vi "Differential Pressure Release Valve Test SAA.vi"(8 "error in (no error)":errorcluster, 10 "Model in":refnum<class "Model.lvclass">, 11 "Test Actuator State in":refnum<class "Test Actuator State.lvclass">) -> (0 "error out":errorcluster, 1 "Pass":bool, 2 "Model out":refnum<class "Model.lvclass">, 3 "Test Actuator State out":refnum<class "Test Actuator State.lvclass">)   [LabVIEW 2016, in "Test Actuator State.lvclass"]
uses:
  Test Actuator State.lvclass
  Model/Model/Model.lvclass
  Model/Model/Model.lvclass/Model.ctl
  Typedefs/ActuatorSetPoints.ctl
  <vilib>/Platform/TimedLoop/XDataNode/timing_clust.ctl
  <vilib>/Platform/TimedLoop/XDataNode/nitl_modes.ctl
  <vilib>/Platform/TimedLoop/XDataNode/wakeup.ctl
  <vilib>/platform/TimedLoop/XDataNode/XDataNode.xnode
  Typedefs/FAMT Typedefs.lvlib
  <vilib>/Platform/TimedLoop/XDataNode/XDNodeRunTimeDep.lvlib
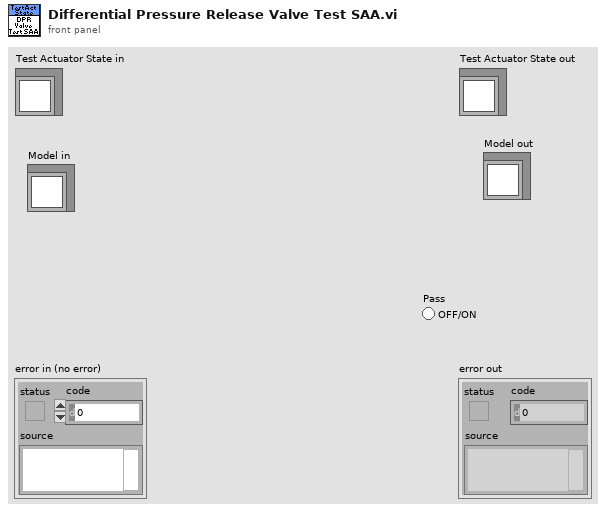
[diagram p1: front panel]
types:
  T1 = typedef "FAMT Typedefs.lvlib/DifferentialPressureReleaseValveTestSettings.ctl" = cluster{"Max Over Force (N)":dbl, "Max Moment (NM)":dbl, "Process Time (s)":dbl, "Sample Time (s)":dbl}
  T2 = typedef "FAMT Typedefs.lvlib/ForcePair.ctl" = cluster{"Axial Force":dbl, "Lateral Force":dbl}
  T3 = typedef "FAMT Typedefs.lvlib/FullForceScanSettings.ctl" = cluster{"Force Tolerance (N)":dbl, "DAA Force Set Points":T2[], "Process Time (s)":dbl, "Sample Time (s)":dbl, "Max Moment (NM)":dbl, "SAA Force Set Points":T2[]}
  T4 = typedef "FAMT Typedefs.lvlib/ActuatorSetPoints.ctl" = cluster{"Axial Force":dbl, "Lateral Force":dbl, "FC1 Force":dbl, "FC2 Force":dbl}
  T5 = typedef "XDNodeRunTimeDep.lvlib/timing_clust.ctl" = cluster{"Expected End [f-1]":u64, "Actual End [f-1]":u64, "Finished Late? [f-1]":bool, "Expected End [i-1]":u64, "Actual End [i-1]":u64, "Finished Late? [i-1]":bool, "Expected Start [i]":u64, "Actual Start [i]":u64, "Expected Start [f]":u64, "Actual Start [f]":u64, "Source Name":string, "Structure Name":string, "Period":i64, "Deadline":i64, "Offset":i64, "Start":i64, "Priority":i32, "Timeout":i32, "Mode":T6, "Wakeup Reason":T7, "Error":errorcluster, "Source Type":string, "Secondary Source Type":string, "Global End Time":u64, "Global Start Time":u64, "Frame Duration":u64, "Iteration Duration":u64, "Assigned CPU":i32, "I/O Scan Engine Mode":u32}
  T6 = typedef "XDNodeRunTimeDep.lvlib/nitl_modes.ctl" = enum32{"No Change", "Process missed periods, maintain original phase", "Discard missed periods, maintain original phase", "Process missed periods, ignore original phase", "Discard missed periods, ignore original phase"}
  T7 = typedef "XDNodeRunTimeDep.lvlib/wakeup.ctl" = enum32{"Normal", "Aborted", "Asynchronous wakeup", "Timing source error", "Timed loop error", "Timeout"}
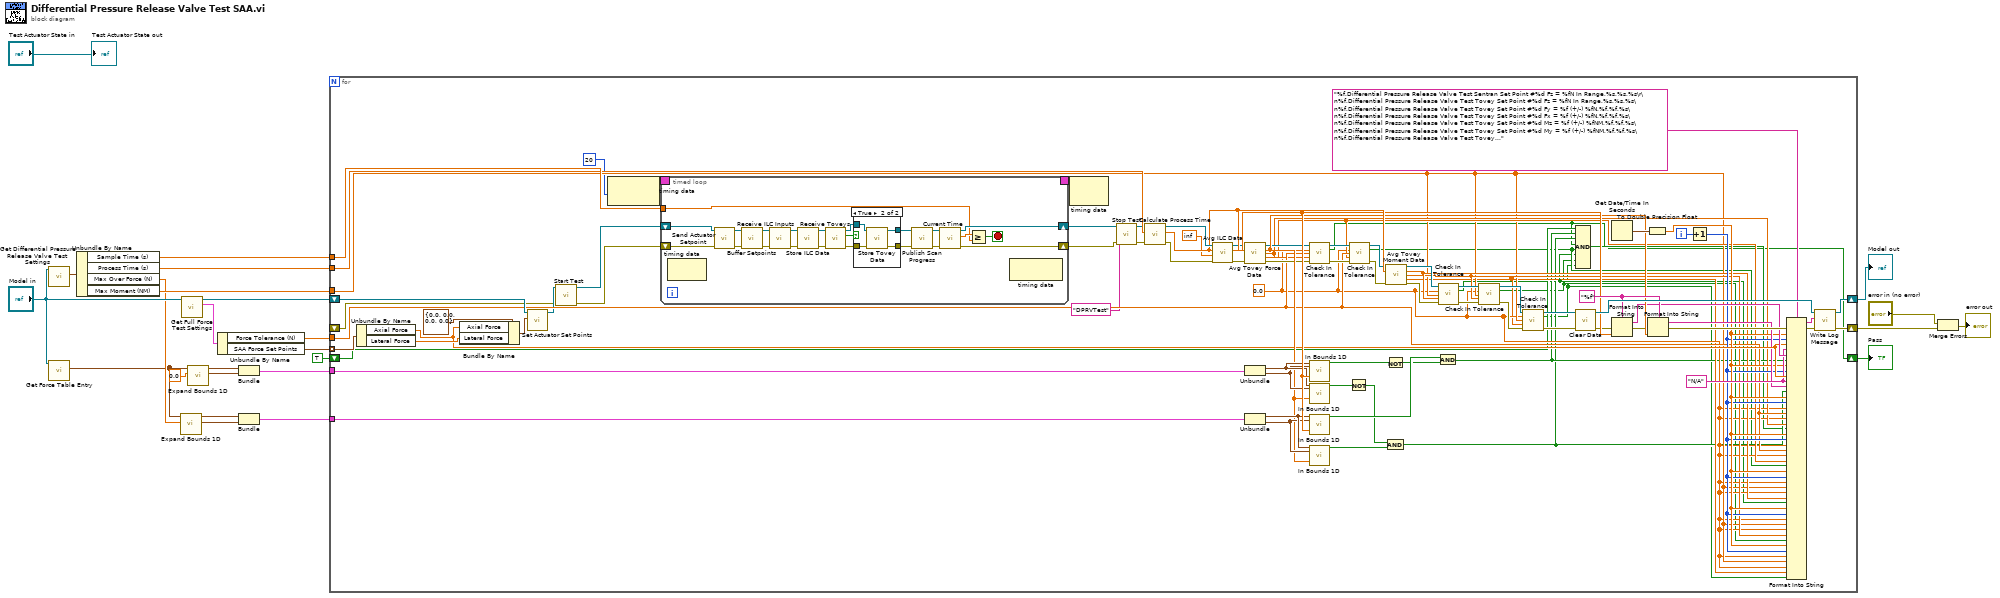
[diagram p0: block diagram]
diagram:
  n1 = call-dynamic "Get Differential Pressure Release Valve Test Settings.vi"("Model in"="Model in") -> ("Differential Pressure Release Valve Test Settings"=w14:T1)  [unwired: 9 in, 1 out]
  n2 = call "Get Force Table Entry.vi"("Model in"="Model in") -> ("Entry"=w8:T2[])  [unwired: 8 in, 2 out]
  n3 = Unbundle By Name(w14) -> ("Sample Time (s)"=w23:dbl, "Process Time (s)"=w22:dbl, "Max Over Force (N)"=w13:dbl, "Max Moment (NM)"=w17:dbl)
  n4 = call "Expand Bounds 1D.vi"("Tolerance (N)"=w13, "Entry"=w8) -> ("Bottom"=w10:T2, "Top"=w11:T2)  [unwired: 8 in]
  n5 = call "Get Full Force Test Settings.vi"("Model in"="Model in") -> ("Full Force Test Settings"=w16:T3, "Model out"=w24:refnum<class "Model.lvclass">)  [unwired: 9 in]
  n6 = call "Expand Bounds 1D.vi"("Tolerance (N)"=0.0, "Entry"=w8) -> ("Bottom"=w5:T2, "Top"=w6:T2)  [unwired: 8 in]
  n7 = Unbundle By Name(w16) -> ("Force Tolerance (N)"=w3:dbl, "SAA Force Set Points"=w12:T2[])
  n8 = Bundle("Top"=w6, "Bottom"=w5) -> (w4:cluster{"Top":T2, "Bottom":T2})  [unwired: 1 in]
  n9 = Bundle("Top"=w11, "Bottom"=w10) -> (w9:cluster{"Top":T2, "Bottom":T2})  [unwired: 1 in]
  n10 = for {
    tunnel: w12 -> [w104] mode=indexing
    shift-right: [w109] -> w19
    shift-left: w24 -> [w112]
    tunnel: w23 -> [w111]
    tunnel: w22 -> [w100]
    shift-right: [w101] -> w18
    shift-left: _ -> [w42]
    tunnel: w17 -> [w50]
    tunnel: w9 -> [w85]
    tunnel: w4 -> [w84]
    tunnel: w3 -> [w55]
    shift-right: [w27] -> w1
    shift-left: TRUE -> [w35]
    i -> [w106]
    w63 = "N/A" ("input 5")
    w79 = "%f" ("format string")
    w49 = 0.0
    n11 = Unbundle By Name(w104) -> ("Axial Force"=w64:dbl, "Lateral Force"=w80:dbl)
    n12 = Bundle By Name(cluster=T4 {"Axial Force"=0.0, "Lateral Force"=0.0, "FC1 Force"=0.0, "FC2 Force"=0.0} ("Actuator Set Points"), "Axial Force"=w64, "Lateral Force"=w80) -> (w105:T4)
    n13 = call "Set Actuator Set Points.vi"("Actuator Set Points"=w105, "Model in"=w112) -> ("Model out"=w43:refnum<class "Model.lvclass">)  [unwired: 9 in]
    n14 = call "Start Test.vi"("error in (no error)"=w42, "Model in"=w43) -> ("error out"=w41:errorcluster, "Model out"=w40:refnum<class "Model.lvclass">)  [unwired: 8 in]
    n15 = node-c288(i64 20 ("Period")) -> (w46:T5)
    n16 = timed-loop {
      shift-right: [w131] -> w39
      shift-left: w40 -> [w135]
      shift-right: [w130] -> w37
      shift-left: w41 -> [w133]
      tunnel: w111 -> [w128]
      timing: w46 -> [_]
      timing-out: [_] -> w45
      stop <- w127 stop-if-true
      n17 = node-c288() -> ()  [unwired: 1 in, 1 out]
      n18 = call "Send Actuator Setpoint.vi"("error in (no error)"=w133, "Model in"=w135) -> ("error out"=w115:errorcluster, "Model out"=w117:refnum<class "Model.lvclass">)  [unwired: 8 in]
      n19 = call "Buffer Setpoints.vi"("error in (no error)"=w115, "Model in"=w117) -> ("error out"=w114:errorcluster, "Model out"=w116:refnum<class "Model.lvclass">)  [unwired: 8 in]
      n20 = call "Receive ILC Inputs.vi"("error in (no error)"=w114, "Model in"=w116) -> ("error out"=w132:errorcluster, "Model out"=w134:refnum<class "Model.lvclass">)  [unwired: 8 in]
      n21 = call "Store ILC Data.vi"("error in (no error)"=w132, "Model in"=w134) -> ("error out"=w125:errorcluster, "Model out"=w126:refnum<class "Model.lvclass">)  [unwired: 8 in]
      n22 = call "Receive Toveys.vi"("error in (no error)"=w125, "Model in"=w126) -> ("error out"=w123:errorcluster, "Data Received"=w122:bool, "Model out"=w124:refnum<class "Model.lvclass">)  [unwired: 7 in]
      n23 = case shown="True" w122 {
        tunnel: w124 -> [w139 w143]
        tunnel: w123 -> [w138 w142]
        tunnel: [w138 w141] -> w118
        tunnel: [w139 w140] -> w121
        frame False {
        }
        frame True {
          n24 = call "Store Tovey Data.vi"("error in (no error)"=w142, "Model in"=w143) -> ("error out"=w141:errorcluster, "Model out"=w140:refnum<class "Model.lvclass">)  [unwired: 8 in]
        }
      }
      n25 = call "Publish Scan Progress.vi"("error in (no error)"=w118, "Model in"=w121) -> ("error out"=w119:errorcluster, "Model out"=w120:refnum<class "Model.lvclass">)  [unwired: 8 in]
      n26 = call "Current Time.vi"("error in (no error)"=w119, "Model in"=w120) -> ("error out"=w130:errorcluster, "Time"=w129:dbl, "Model out"=w131:refnum<class "Model.lvclass">)  [unwired: 7 in]
      n27 = Greater Or Equal?(x=w129, y=w128) -> (x >= y?=w127:bool)
      n28 = node-c288() -> ()  [unwired: 1 in, 1 out]
    }
    n29 = node-c288(w45) -> ()  [unwired: 1 out]
    n30 = call "Stop Test.vi"("error in (no error)"=w37, "Test"="DPRVTest", "Model in"=w39) -> ("error out"=w36:errorcluster, "Model out"=w38:refnum<class "Model.lvclass">)  [unwired: 7 in]
    n31 = call "Calculate Process Time.vi"("error in (no error)"=w36, "Seconds"=w100, "Model in"=w38) -> ("error out"=w98:errorcluster, "Time"=w97:dbl, "Model out"=w99:refnum<class "Model.lvclass">)  [unwired: 6 in]
    n32 = call "Avg ILC Data.vi"("error in (no error)"=w98, "Before This Time"=inf, "After This Time"=w97, "Model in"=w99) -> ("error out"=w96:errorcluster, "Fz"=w78:dbl, "Model out"=w69:refnum<class "Model.lvclass">)  [unwired: 4 in, 1 out]
    n33 = call "Avg Tovey Force Data.vi"("Model in"=w69, "After This Time"=w97, "error in (no error)"=w96) -> ("Model out"=w59:refnum<class "Model.lvclass">, "Fz"=w73:dbl, "Fy"=w54:dbl, "Fx"=w53:dbl, "error out"=w57:errorcluster)  [unwired: 8 in]
    n34 = Unbundle(w84) -> ("Top"=w75:T2, "Bottom"=w74:T2)
    n35 = Unbundle(w85) -> ("Top"=w77:T2, "Bottom"=w76:T2)
    n36 = call "Check In Tolerance.vi"("Model in"=w59, "Expected"=w49, "Tolerance"=w55, "Actual"=w54, "error in (no error)"=w57) -> ("Model out"=w58:refnum<class "Model.lvclass">, "Pass"=w32:bool, "error out"=w56:errorcluster)  [unwired: 8 in]
    n37 = call "In Bounds 1D.vi"("Top"=w75, "Bottom"=w74, "Axial"=w78) -> ("InBounds"=w83:bool)  [unwired: 16 in]
    n38 = call "In Bounds 1D.vi"("Top"=w75, "Bottom"=w74, "Axial"=w73) -> ("InBounds"=w72:bool)  [unwired: 16 in]
    n39 = call "In Bounds 1D.vi"("Top"=w77, "Bottom"=w76, "Axial"=w78) -> ("InBounds"=w82:bool)  [unwired: 16 in]
    n40 = call "In Bounds 1D.vi"("Top"=w77, "Bottom"=w76, "Axial"=w73) -> ("InBounds"=w70:bool)  [unwired: 16 in]
    n41 = Not(x=w72) -> (.not. x?=w71:bool)
    n42 = call "Check In Tolerance.vi"("Model in"=w58, "Expected"=w49, "Tolerance"=w55, "Actual"=w53, "error in (no error)"=w56) -> ("Model out"=w94:refnum<class "Model.lvclass">, "Pass"=w31:bool, "error out"=w95:errorcluster)  [unwired: 8 in]
    n43 = Not(x=w83) -> (.not. x?=w81:bool)
    n44 = And(x=w71, y=w70) -> (x .and. y?=w33:bool)
    n45 = call "Avg Tovey Moment Data.vi"("Model in"=w94, "After This Time"=w97, "error in (no error)"=w95) -> ("Model out"=w93:refnum<class "Model.lvclass">, "Mz"=w52:dbl, "My"=w51:dbl, "Mx"=w48:dbl, "error out"=w92:errorcluster)  [unwired: 8 in]
    n46 = And(x=w82, y=w81) -> (x .and. y?=w34:bool)
    n47 = call "Check In Tolerance.vi"("Model in"=w93, "Expected"=w49, "Tolerance"=w50, "Actual"=w52, "error in (no error)"=w92) -> ("Model out"=w91:refnum<class "Model.lvclass">, "Pass"=w30:bool, "error out"=w88:errorcluster)  [unwired: 8 in]
    n48 = call "Check In Tolerance.vi"("Model in"=w91, "Expected"=w49, "Tolerance"=w50, "Actual"=w51, "error in (no error)"=w88) -> ("Model out"=w90:refnum<class "Model.lvclass">, "Pass"=w29:bool, "error out"=w87:errorcluster)  [unwired: 8 in]
    n49 = call "Check In Tolerance.vi"("Model in"=w90, "Expected"=w49, "Tolerance"=w50, "Actual"=w48, "error in (no error)"=w87) -> ("Model out"=w89:refnum<class "Model.lvclass">, "Pass"=w28:bool, "error out"=w86:errorcluster)  [unwired: 8 in]
    n50 = call "Clear Data.vi"("error in (no error)"=w86, "Model in"=w89) -> ("error out"=w68:errorcluster, "Model out"=w110:refnum<class "Model.lvclass">)  [unwired: 8 in]
    n51 = Compound Arithmetic op=AND(w35, w34, w33, w32, w31, w30, w29, w28) -> (w27:bool)
    n52 = Get Date/Time In Seconds() -> (seconds since 1Jan1904=w107:timestamp)
    n53 = Format Into String(format string=w79, error in=w68, w78) -> (resulting string=w65:string, error out=w67:errorcluster)  [unwired: 1 in]
    n54 = To Double Precision Float(number=w107) -> (double precision float=w61:dbl)
    n55 = Format Into String(format string=w79, error in=w67, w73) -> (resulting string=w62:string, error out=w66:errorcluster)  [unwired: 1 in]
    n56 = Increment(x=w106) -> (x+1=w60:i32)
    n57 = Format Into String(format string="%f,Differential Pressure Release Valve Test Sentran Set Point #%d Fz = %fN In Range,%s,%s,%s\r\n%f,Differential Pressure Release Valve Test Tovey Set Point #%d Fz = %fN In Range,%s,%s,%s\n%f,Differential Pressure Release Valve Test Tovey Set Point #%d Fy = %f (+/-) %fN,%f,%f,%s\n%f,Differential Pressure Release Valve Test Tovey Set Point #%d Fx = %f (+/-) %fN,%f,%f,%s\n%f,Differential Pressure Release Valve Test Tovey Set Point #%d Mz = %f (+/-) %fNM,%f,%f,%s\n%f,Differential Pressure Release Valve Test Tovey Set Point #%d My = %f (+/-) %fNM,%f,%f,%s\n%f,Differential Pressure Release Valve Test Tovey Set Point #%d Mx = %f (+/-) %fNM,%f,%f,%s\n", error in=w66, w61, w60, w64, w63, w65, w34, w61, w60, w64, w63, w62, w33, w61, w60, w49, w55, w49, w54, w32, w61, w60, w49, w55, w49, w53, w31, w61, w60, w49, w50, w49, w52, w30, w61, w60, w49, w50, w49, w51, w29, w61, w60, w49, w50, w49, w48, w28) -> (resulting string=w103:string, error out=w102:errorcluster)  [unwired: 1 in]
    n58 = call "Write Log Message.vi"("error in (no error)"=w102, "Message"=w103, "Model in"=w110) -> ("error out"=w101:errorcluster, "Model out"=w109:refnum<class "Model.lvclass">)  [unwired: 7 in]
  }
  "Model out" <- w19
  "Pass" <- w1
  n59 = Merge Errors("error in (no error)", w18) -> (→"error out":errorcluster)
  "Test Actuator State out" <- "Test Actuator State in"
